vi "RTI Connext DDS Read String.vi"() -> ()   [LabVIEW 2021]
doc: "Shows how to subscribe (read) to a string using RTI Connext DDS. It was created using the simple read/write example in the Getting Started Guide (<LabVIEW folder>/help/RTI DDS Toolkit/RTI_DDS_Toolkit_GettingStarted.pdf)."
uses:
  <vilib>/RTI DDS Toolkit/VIs/SimpleCreateReader_String.vi
  <vilib>/RTI DDS Toolkit/VIs/Read_String.vi
  <vilib>/RTI DDS Toolkit/VIs/Advanced Create Reader.vi
  <vilib>/RTI DDS Toolkit/VIs/AdvancedCreateReader_String.vi
  <vilib>/RTI DDS Toolkit/Library/LVDDS_library.lvlib
panel:
  in  "Stop Reading":bool
  out "Text":string
  in  "error in (no error)":errorcluster
  # "Overview: Demonstrate how to subscribe to and read a String type using Connext DDS.\nRequirements: RTI DDS Toolkit\nInstructions:\n1. Run the VI.\n2. Run the RTI Connext DDS Write String.vi example.\n3. Check whether you are receiving the correct information published by the RTI Connext DDS Write String.vi example.\n\nMore information about this and other examples can be found in RTI_DDS_Toolkit_GettingStarted.pdf"
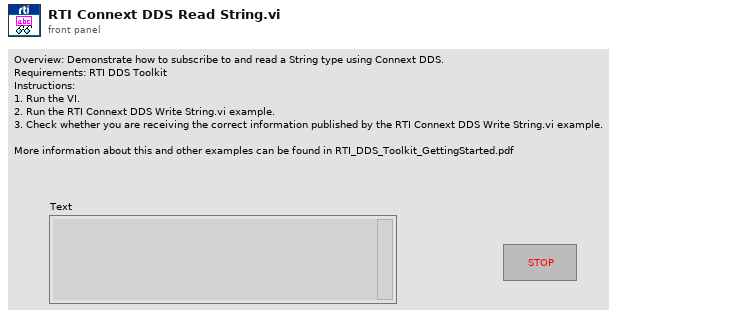
[diagram p1: front panel]
types:
  T1 = typedef "LVDDS_library.lvlib/DDS Sample Info.ctl" = cluster{"DDS_SampleStateKind":enum32{"DDS_INVALID_SAMPLE_STATE", "DDS_READ_SAMPLE_STATE", "DDS_NOT_READ_SAMPLE_STATE"}, "DDS_ViewStateKind":enum32{"DDS_INVALID_SAMPLE_STATE", "DDS_NEW_VIEW_STATE", "DDS_NOT_NEW_VIEW_STATE"}, "DDS_InstanceStateKind":enum32{"DDS_INVALID_STATE", "DDS_ALIVE_INSTANCE_STATE", "DDS_NOT_ALIVE_DISPOSED_INSTANCE_STATE", "", "DDS_NOT_ALIVE_NO_WRITERS_INSTANCE_STATE"}, "sec":i32, "nanosec":u32, "valid_data":bool}
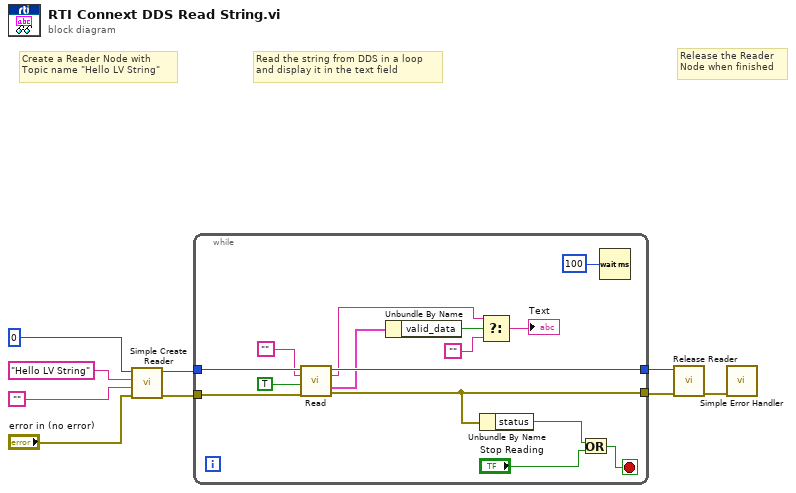
[diagram p0: block diagram]
diagram:
  # "Release the Reader\nNode when finished"
  # "Read the string from DDS in a loop \nand display it in the text field"
  # "Create a Reader Node with \nTopic name \"Hello LV String\""
  n1 = call-poly <vilib>:"Simple Create Reader.vi"("error in"="error in (no error)", "Type"="", "Topic Name"="Hello LV String", "Domain Id"=u32 0) -> ("error out"=w3:errorcluster, "DDS Object Ref"=w2:u64)  [unwired: 6 in]
  n2 = while {
    tunnel: w3 -> [w17]
    tunnel: [w19] -> w9
    tunnel: [w24] -> w8
    tunnel: w2 -> [w22]
    stop <- w20 stop-if-true
    n3 = call-poly <vilib>:"Read.vi"("DDS Object Ref in"=w22, "Query Condition"="", "Only New Samples"=TRUE ("Read All Samples"), "error in (no error)"=w17) -> ("DDS Object Ref out"=w24:u64, "Data"=w12:string, "DDS Sample Info"=w14:T1, "error out"=w19:errorcluster)  [unwired: 7 in, 1 out]
    n4 = Unbundle By Name(w14) -> ("valid_data"=w13:bool)
    n5 = Unbundle By Name(w19) -> ("status"=w21:bool)
    n6 = Select(t=w12, s=w13, f="") -> (s? t:f=→"Text":string)
    n7 = Or(x=w21, y="Stop Reading") -> (x .or. y?=w20:bool)
    n8 = Wait (ms)(milliseconds to wait=u32 100 ("millisecond multiple")) -> ()  [unwired: 1 out]
  }
  n9 = call <vilib>:"Release Reader.vi"("error in (no error)"=w9, "DDS Object Ref"=w8) -> ("error out"=w7:errorcluster)  [unwired: 9 in]
  n10 = call <vilib>:"Simple Error Handler.vi"("error in (no error)"=w7) -> ()  [unwired: 4 in, 5 out]
